vi "Xeryon Axis SendCommand.vi"(3 "error in (no error)":errorcluster, 4 "Feedback?":bool, 5 "Stage":string, 6 "Axis Command":T1={"Command"=enum."Exit", "Data to send"=""}) -> (0 "error out":errorcluster)   [LabVIEW 2014]
uses:
  Xeryon Axis command.ctl
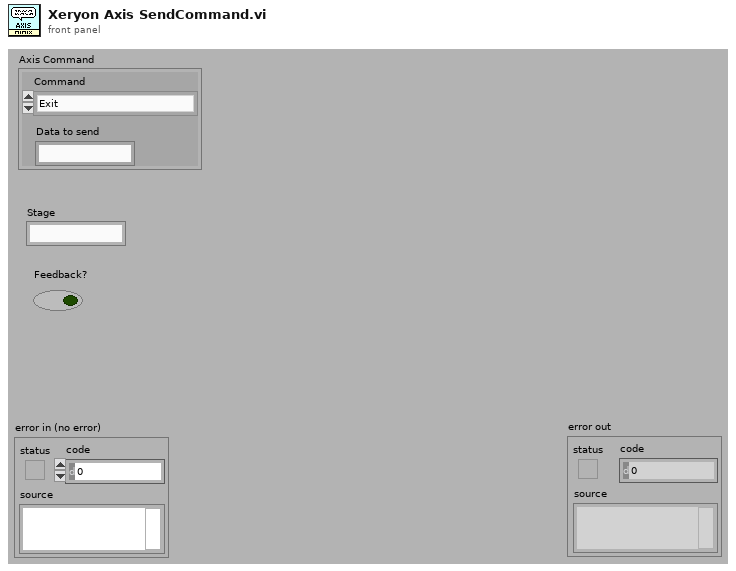
[diagram p1: front panel]
types:
  T1 = typedef "Xeryon Axis command.ctl" = cluster{"Command":enum16{"Reset", "Zero output", "Go home", "Find index", "Scan -X", "Scan +X", "Scan Stop", "Step -X", "Step +X", "Set DPOS", "Stop", "Continue", "Desired speed", "Apply settings file", "Exit", "Reset encoder", "Recover", "Save"}, "Data to send":string}
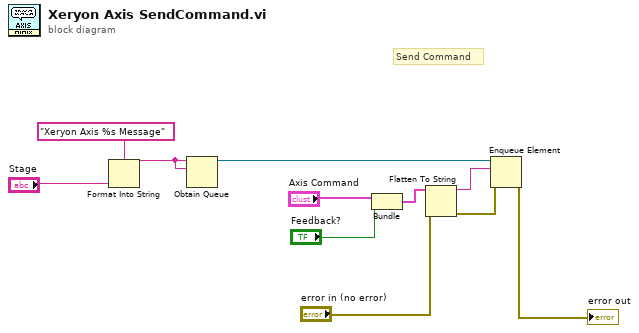
[diagram p0: block diagram]
diagram:
  # "Send Command"
  n1 = Format Into String(format string="Xeryon Axis %s Message" ("name (unnamed)"), "Stage") -> (resulting string=w3:string)  [unwired: 2 in, 1 out]
  n2 = Obtain Queue(name (unnamed)=w3, element data type=w3) -> (queue out=w8:refnum<queue>)  [unwired: 3 in, 2 out]
  n3 = Bundle("Axis Command"="Axis Command", "Feedback?"="Feedback?") -> (w10:cluster{"Axis Command":T1, "Feedback?":bool})  [unwired: 1 out]
  n4 = Flatten To String(anything=w10, error in (no error)="error in (no error)") -> (data string=w2:string, error out=w6:errorcluster)  [unwired: 3 out]
  n5 = Enqueue Element(queue=w8, element=w2, error in (no error)=w6) -> (error out=→"error out":errorcluster)  [unwired: 3 out]
